vi "Get Horizontal-Vertical Cursor Position.vi"(8 "error in (no error)":errorcluster, 10 "Cursor":T1, 11 "VISA resource name":refnum<visa-resource-name>) -> (0 "error out":errorcluster, 2 "Position":dbl format="%.9f", 3 "VISA resource name out":refnum<visa-resource-name>)   [LabVIEW 2018, in "DPO4104.lvlib" / "DPO4104.lvclass"]
doc: "This VI sends commands to retrieve the cursors' position."
uses:
  DPO4104.lvclass
  PPLs/Oscilloscope/Parent/Oscilloscope.lvlibp/Custom Controls/Select Cursor.ctl
  <instrlib>/Tektronix DPO MSO 2000 4000 Series/Tektronix DPO MSO 2000 4000 Series.lvlib
  PPLs/Oscilloscope/Parent/Oscilloscope.lvlibp
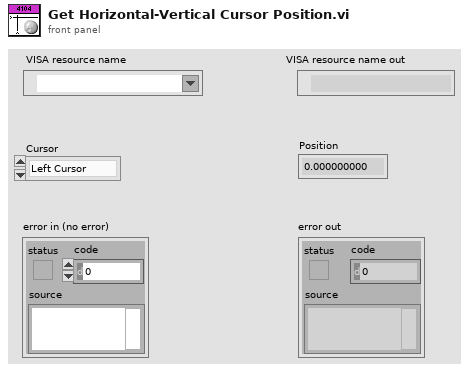
[diagram p1: front panel]
types:
  T1 = typedef "Oscilloscope.lvlibp/Select Cursor.ctl" = enum16{"Left Cursor", "Right Cursor", "Top Cursor", "Bottom Cursor"}
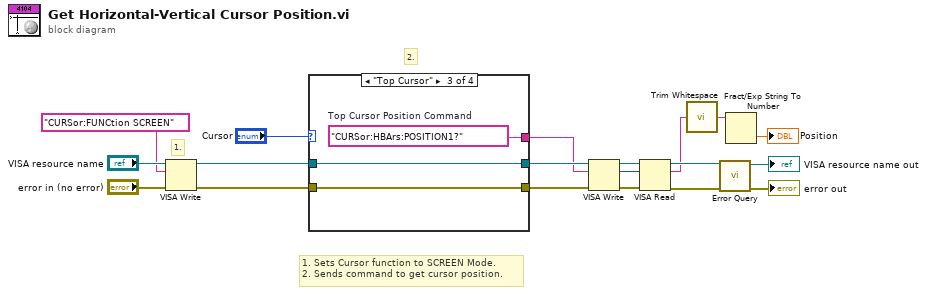
[diagram p0: block diagram]
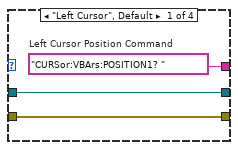
[diagram p2: hidden frame]
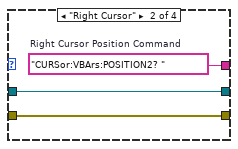
[diagram p3: hidden frame]
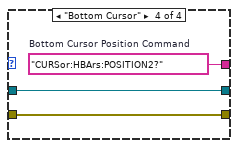
[diagram p4: hidden frame]
diagram:
  # "1. Sets Cursor function to SCREEN Mode.\n2. Sends command to get cursor position."
  # "2."
  # "1."
  n1 = VISA Write(VISA resource name="VISA resource name", write buffer="CURSor:FUNCtion SCREEN", error in (no error)="error in (no error)") -> (VISA resource name out=w2:refnum<visa-resource-name>, error out=w1:errorcluster)  [unwired: 1 out]
  n2 = case shown="\"Top Cursor\"" "Cursor" {
    tunnel: [w22 w25 w28 w31] -> w4
    tunnel: w2 -> [w21 w24 w27 w30]
    tunnel: w1 -> [w20 w23 w26 w29]
    tunnel: [w21 w24 w27 w30] -> w6
    tunnel: [w20 w23 w26 w29] -> w5
    frame "Left Cursor", Default {
      w22 = "CURSor:VBArs:POSITION1? "  # Left Cursor Position Command
    }
    frame "Right Cursor" {
      w25 = "CURSor:VBArs:POSITION2? "  # Right Cursor Position Command
    }
    frame "Top Cursor" {
      w28 = "CURSor:HBArs:POSITION1?"  # Top Cursor Position Command
    }
    frame "Bottom Cursor" {
      w31 = "CURSor:HBArs:POSITION2?"  # Bottom Cursor Position Command
    }
  }
  n3 = VISA Write(VISA resource name=w6, write buffer=w4, error in (no error)=w5) -> (VISA resource name out=w19:refnum<visa-resource-name>, return count=w3:u32, error out=w18:errorcluster)
  n4 = VISA Read(VISA resource name=w19, byte count=w3, error in (no error)=w18) -> (VISA resource name out=w15:refnum<visa-resource-name>, read buffer=w11:string, error out=w14:errorcluster)  [unwired: 1 out]
  n5 = call <vilib>:"Trim Whitespace.vi"("string"=w11) -> ("trimmed string"=w13:string)  [unwired: 1 in]
  n6 = call <instrlib>:"Error Query.vi"("error in (no error)"=w14, "VISA resource name"=w15) -> ("error out"=→"error out":errorcluster, "VISA resource name out"=→"VISA resource name out":refnum<visa-resource-name>)  [unwired: 6 in, 2 out]
  n7 = Fract/Exp String To Number(string=w13) -> (number=→"Position":dbl)  [unwired: 3 in, 1 out]
